vi "Read Voltage.vi"(4 "에러 입력(에러 없음)":errorcluster) -> (0 "에러 출력":errorcluster, 3 "전압":dbl format="%.2f")   [LabVIEW 2010]
doc: "이 VI는 DAQ 보드로부터 전압 값을 읽어오는 시뮬레이션을 합니다. 이 VI를 사용하여 교육과정의 모든 온도 읽기 연습 문제에 나오는 DAQ 어시스턴트 익스프레스 VI를 대체합니다. 이 VI는 모든 (데모) 연습문제에서 SubVI로 사용됩니다."
panel:
  in  "읽기":dbl[](array[numeric])=[163.0, 163.0, 163.0, 163.0, 163.0, 163.0, 165.0, 169.0, 172.0, 173.0, 172.0, 172.0, 171.0, 171.0, 174.0, 176.0, 177.0, 178.0, 178.0, 179.0, 178.0, 177.0, 176.0, 175.0, 175.0, 174.0, 173.0, 172.0, 172.0, 172.0, 172.0, 172.0, 171.0, 171.0, 170.0, 170.0, 170.0, 172.0, 173.0, 174.0, 175.0, 177.0, 178.0, 178.0, 178.0, 177.0, 176.0, 175.0, 176.0, 178.0, 179.0, 180.0, 179.0, 178.0, 178.0, 176.0, 176.0, 176.0, 174.0, 174.0, 174.0, 173.0, 173.0, 175.0, 176.0, 178.0, 178.0, 177.0, 176.0, 175.0, 175.0, 174.0, 174.0, 173.0, 173.0, 172.0, 172.0, 171.0, 171.0, 170.0, 170.0, 170.0, 170.0, 170.0, 170.0, 170.0, 169.0, 166.0, 167.0, 169.0, 170.0, 169.0, 168.0, 168.0, 168.0, 168.0, 167.0, 167.0, 167.0, 167.0] format="%.2f"
  # "*이 VI는 디바이스 1, 채널 0에서\n전압을 읽고 온도로 변환하기 위해\n그 신호에 100을 스케일한\nVI의 데모 버전입니다.*"
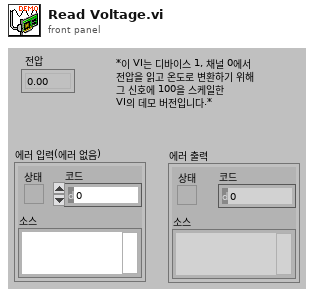
[diagram p1: front panel]
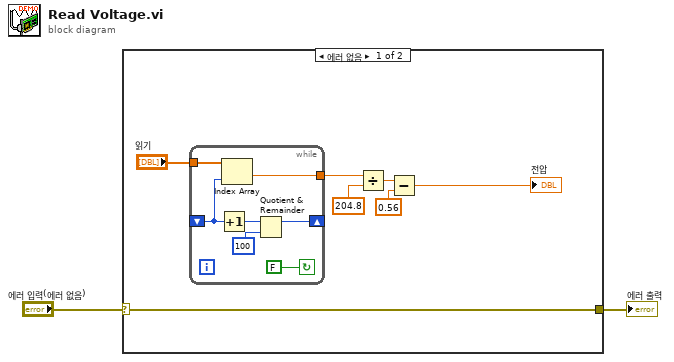
[diagram p0: block diagram]
diagram:
  n1 = case shown="에러 없음" "에러 입력(에러 없음)" {
    selector: "에러 입력(에러 없음)" -> [w4 w17]
    tunnel: [w4 w17] -> w1
    frame No Error {
      n2 = while {
        tunnel: "읽기" -> [w11]
        tunnel: [w12] -> w7
        shift-left: _ -> [w16]
        shift-right: [w13] -> _
        stop <- FALSE continue-if-true
        n3 = Increment(x=w16) -> (x+1=w15:i32)
        n4 = Index Array(array=w11, index=w16) -> (element=w12:dbl)
        n5 = Quotient & Remainder(x=w15, y=100) -> (x-y*floor(x/y)=w13:i32)  [unwired: 1 out]
      }
      n6 = Divide(x=w7, y=204.8) -> (x/y=w6:dbl)
      n7 = Subtract(x=w6, y=0.56) -> (x-y=→"전압":dbl)
    }
    frame Error {
    }
  }
  "에러 출력" <- w1
